vi "niRFUtil LCAPI Copy 1D Array (2 DBL).vi"(0 "Source0 1D Array (DBL)":dbl[](array[numeric]) format="%.2f", 5 "Source1 1D Array (DBL)":dbl[](array[numeric]) format="%.2f", 11 "error in (no error)":errorcluster, 12 "Data Copy Descriptor":u64) -> (4 "Source0 Out":dbl[](array[numeric]) format="%.2f", 6 "Source1 Out":dbl[](array[numeric]) format="%.2f", 15 "error out":errorcluster)   [LabVIEW 2015, in "niRFUtil.lvlib"]
uses:
  niRFUtil.lvlib
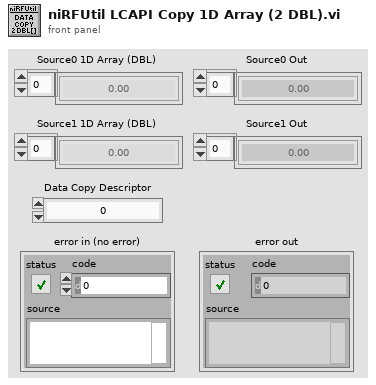
[diagram p1: front panel]
types:
  T1 = cluster{"status":bool, "return type":i32, "errorString":string}
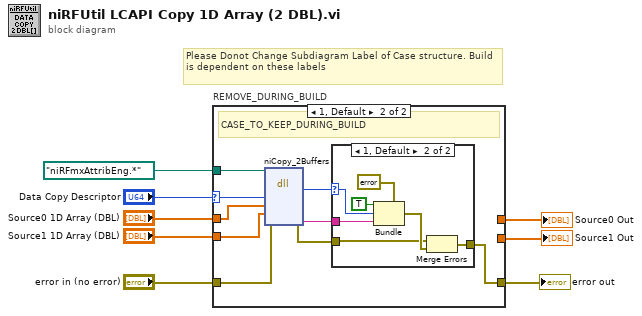
[diagram p0: block diagram]
diagram:
  # "Please Donot Change Subdiagram Label of Case structure. Build is dependent on these labels"
  n1 = case "REMOVE_DURING_BUILD" shown="1, Default" "Data Copy Descriptor" {
    selector: "Data Copy Descriptor" -> [_ w13]
    tunnel: [w9 w20] -> w8
    tunnel: "error in (no error)" -> [w9 w19]
    tunnel: "Source0 1D Array (DBL)" -> [w11 w18]
    tunnel: "Source1 1D Array (DBL)" -> [w10 w17]
    tunnel: [w11 _] -> w3
    tunnel: [w10 _] -> w2
    tunnel: path "niRFmxAttribEng.*" ("path in") -> [_ w12]
    frame 0 {
      # "Developement"
    }
    frame 1, Default {
      # "CASE_TO_KEEP_DURING_BUILD"
      n2 = dll-call lib="niRFmxAttribEng.*" fn="niCopy_2Buffers"(path in=w12, error in=w19, "dataCopyDescriptor"=w13, "source0"=w18, "source1"=w17) -> (error out=w14:errorcluster, "return type"=w16:i32, "errorString"=w15:string)  [unwired: 5 in, 1 out]
      n3 = case shown="1, Default" w16 {
        selector: w16 -> [_ w26]
        tunnel: w15 -> [_ w25]
        tunnel: w14 -> [w21 w23]
        tunnel: [w21 w27] -> w20
        frame 0 {
        }
        frame 1, Default {
          n4 = Bundle(cluster=T1 {"status"=FALSE, "return type"=0, "errorString"=""}, "status"=TRUE, "return type"=w26, "errorString"=w25) -> (w24:T1)
          n5 = Merge Errors(w23, w24) -> (w27:errorcluster)
        }
      }
    }
  }
  "error out" <- w8
  "Source0 Out" <- w3
  "Source1 Out" <- w2
